vi "Wrapper_Destroy_Mod.vi"(8 "error in (no error)":errorcluster caption="entrée d'erreur (pas d'erreur)", 10 "Wrapper":u32) -> (0 "error out":errorcluster caption="sortie d'erreur")   [LabVIEW 2024]
uses:
  OmniDriver32.dll
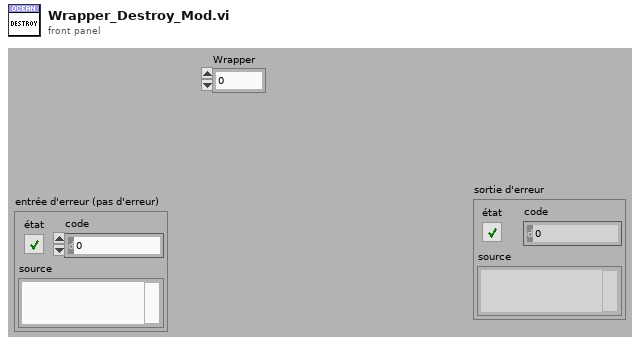
[diagram p1: front panel]
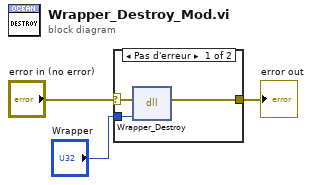
[diagram p0: block diagram]
diagram:
  n1 = case shown="Pas d'erreur" "error in (no error)" {
    selector: "error in (no error)" -> [w5 w7]
    tunnel: "Wrapper" -> [w6 _]
    tunnel: [w4 w7] -> w1
    frame No Error {
      n2 = dll-call lib="OmniDriver32.dll" fn="Wrapper_Destroy" label="Wrapper.Destroy"(error in=w5, "Wrapper"=w6) -> (error out=w4:errorcluster)  [unwired: 3 in, 2 out]
    }
    frame Error {
    }
  }
  "error out" <- w1
